vi "Do.vi"(8 "error in (no error)":errorcluster, 10 "Actor in":refnum<class "Actor.lvclass">, 11 "Add Timestamped Data Msg":refnum<class "Add Timestamped Data Msg.lvclass">) -> (0 "error out":errorcluster, 2 "Actor out":refnum<class "Actor.lvclass">)   [LabVIEW 2018, in "BNT_XtGraph.lvlib" / "Add Timestamped Data Msg.lvclass"]
doc: "This VI delivers the message to the actor by calling the appropriate method(s) on the actor."
uses:
  Add Timestamped Data Msg.lvclass
  <vilib>/ActorFramework/Actor/Actor.lvclass
  BNT_XtGraph/BNT_XtGraph.lvclass
  C:/Program Files (x86)/National Instruments/LabVIEW 2018/vi.lib/ActorFramework/Actor/Actor.lvclass
  Add Timestamped Data Msg.lvclass/Add Timestamped Data Msg.ctl
  CSPP_Core/Messages/CSPP_AsyncCallbackMsg/CSPP_AsyncCallback Msg.lvclass
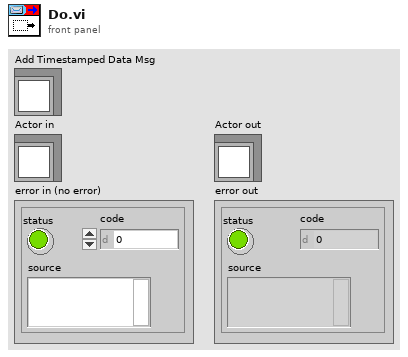
[diagram p1: front panel]
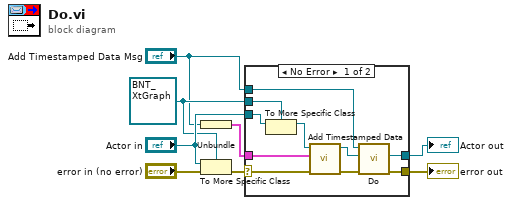
[diagram p0: block diagram]
diagram:
  w3 = refnum<class "BNT_XtGraph.lvclass"> refnum ("Actor in")
  n1 = Unbundle ("Main-Unbundler")("Add Timestamped Data Msg") -> (w1:cluster{"Time Stamp":timestamp, "Value":dbl}[])
  n2 = To More Specific Class(target class=w3, reference="Actor in", error in="error in (no error)") -> (error out=w7:errorcluster)  [unwired: 1 out]
  n3 = case shown="No Error" w7 {
    selector: w7 -> [w18 w20]
    tunnel: [w14 w20] -> w6
    tunnel: [w13 w19] -> w5
    tunnel: "Actor in" -> [w17 w19]
    tunnel: w3 -> [w16 _]
    tunnel: "Add Timestamped Data Msg" -> [w10 _]
    tunnel: w1 -> [w9 _]
    frame No Error {
      n4 = To More Specific Class ("To More Specific Class (internal)")(target class=w16, reference=w17) -> (specific class reference=w15:refnum<class "BNT_XtGraph.lvclass">)  [unwired: 1 in, 1 out]
      n5 = call "Add Timestamped Data.vi"("Error In"=w18, "X-t Value Pairs"=w9, "BNT_XtGraph in"=w15) -> ("Error Out"=w11:errorcluster, "BNT_XtGraph out"=w12:refnum<class "BNT_XtGraph.lvclass">)  [unwired: 7 in]
      n6 = call-parent "Do.vi"("error in (no error)"=w11, "Actor in"=w12, "CSPP_AsyncCallback Msg"=w10) -> ("error out"=w14:errorcluster, "Actor out"=w13:refnum<class "Actor.lvclass">)  [unwired: 7 in]
    }
    frame Error {
    }
  }
  "error out" <- w6
  "Actor out" <- w5
